vi "LED blinker.vi"(8 "error in (no error)":errorcluster, 10 "Color 1":u32(colorbox)=16860, 11 "Color 2":u32(colorbox)=61205) -> ()   [LabVIEW 2019]
uses:
  2020 Robot/Framework/Robot Global Data.vi
panel:
  in  "Color 3":u32(colorbox)=16711680
  in  "y":dbl=2.0 format="%#_13g"
  out "LED Strip":u32[](array[colorbox])
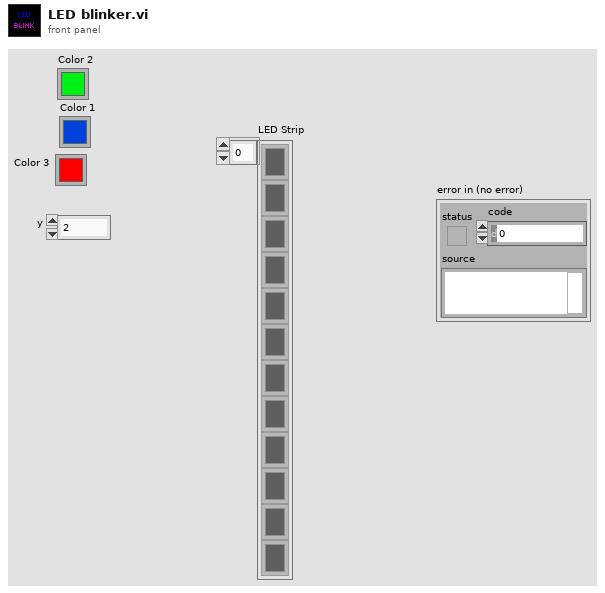
[diagram p1: front panel]
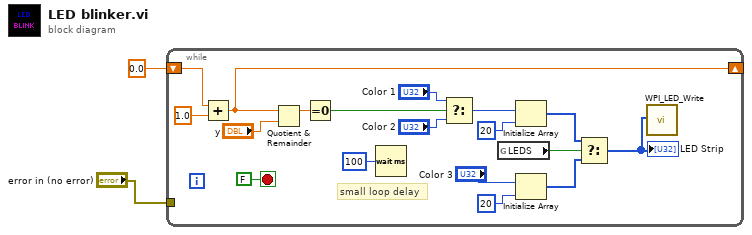
[diagram p0: block diagram]
diagram:
  n1 = while {
    shift-right: [w16] -> _
    shift-left: 0.0 -> [w17]
    tunnel: "error in (no error)" -> [_]
    stop <- FALSE ("x") stop-if-true
    # "small loop delay"
    n2 = Add(x=w17, y=1.0) -> (x+y=w16:dbl)
    n3 = Quotient & Remainder(x=w16, y="y") -> (x-y*floor(x/y)=w14:dbl)  [unwired: 1 out]
    n4 = Equal To 0?(x=w14) -> (x = 0?=w7:bool)
    n5 = Wait (ms)(milliseconds to wait=u32 100) -> ()  [unwired: 1 out]
    n6 = Select(t="Color 1", s=w7, f="Color 2") -> (s? t:f=w4:u32)
    n7 = global read "Robot Global Data.vi" "LEDS"() -> (w11:bool)
    n8 = Initialize Array(w4, 20 ("dimension size")) -> (w10:u32[])
    n9 = Initialize Array("Color 3", 20 ("dimension size")) -> (w9:u32[])
    n10 = Select(t=w10, s=w11, f=w9) -> (s? t:f=w8:u32[])
    "LED Strip" <- w8
    n11 = call <vilib>:"WPI_LED_Write.vi"("Color Array"=w8) -> ()  [unwired: 10 in, 1 out]
  }
